vi "svfa_Spectrum Peak Tone Search and Estimation.vi"   [LabVIEW 2017]
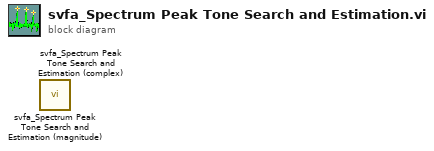
[diagram p0: block diagram]
diagram:
  n1 = call <vilib>:"svfa_Spectrum Peak Tone Search and Estimation (magnitude).vi"() -> ()  [unwired: 9 in, 3 out]
  n2 = call <vilib>:"svfa_Spectrum Peak Tone Search and Estimation (complex).vi"() -> ()  [unwired: 9 in, 3 out]
